vi "Load from File.vi"(5 "File Path (dialog)":path, 11 "Error In":errorcluster) -> (4 "Neural Network Out":T1={"Weigths"=[], "Last Layer Linear"=TRUE, "Add Bias Inputs"=TRUE, "# Inputs"=0, "# Output Neurons/Outputs"=0, "Inputs Scaling"={"X Scaling Vector"=[], "Y Scaling Vector"=[]}, "Outputs Scaling"={"X Scaling Vector"=[], "Y Scaling Vector"=[]}}, 6 "Used Path":path, 10 "Cancelled":bool, 15 "Error Out":errorcluster)   [LabVIEW 2013, in "Super Simple Neural Network.lvlib"]
doc: "This VI loads neural network from a file."
uses:
  Super Simple Neural Network.lvlib
  Types/Neural Network.ctl
  Types/2D Array.ctl
  Types/Scaling Info.ctl
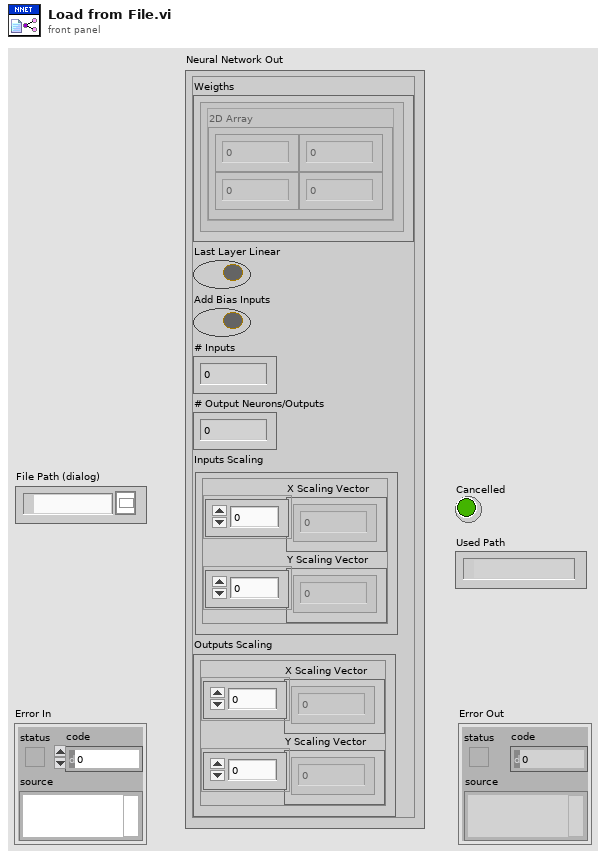
[diagram p1: front panel]
types:
  T1 = typedef "Super Simple Neural Network.lvlib/Neural Network.ctl" = cluster{"Weigths":T2[], "Last Layer Linear":bool, "Add Bias Inputs":bool, "# Inputs":u32, "# Output Neurons/Outputs":u32, "Inputs Scaling":T3, "Outputs Scaling":T3}
  T2 = typedef "Super Simple Neural Network.lvlib/2D Array.ctl" = cluster{"2D Array":dbl[][]}
  T3 = typedef "Super Simple Neural Network.lvlib/Scaling Info.ctl" = cluster{"X Scaling Vector":dbl[], "Y Scaling Vector":dbl[]}
  T4 = enum16{"open", "replace", "create", "open or create", "replace or create", "replace or create with confirmation"}
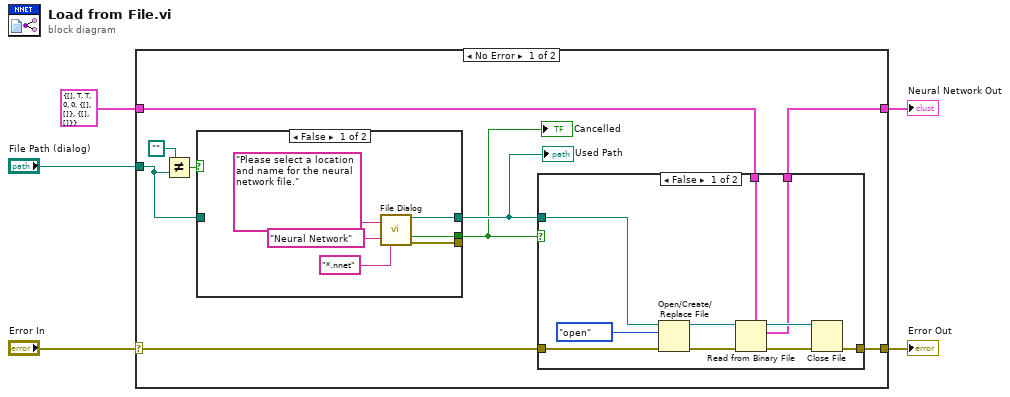
[diagram p0: block diagram]
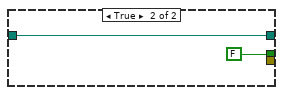
[diagram p3: hidden frame]
diagram:
  n1 = case shown="No Error" "Error In" {
    selector: "Error In" -> [w13 w36]
    tunnel: [w11 w36] -> w4
    tunnel: [w9 w35] -> w2
    tunnel: T1 {"Weigths"=[], "Last Layer Linear"=TRUE, "Add Bias Inputs"=TRUE, "# Inputs"=0, "# Output Neurons/Outputs"=0, "Inputs Scaling"={"X Scaling Vector"=[], "Y Scaling Vector"=[]}, "Outputs Scaling"={"X Scaling Vector"=[], "Y Scaling Vector"=[]}} ("Neural Network In") -> [w12 w35]
    tunnel: "File Path (dialog)" -> [w6 _]
    frame No Error {
      n2 = Not Equal?(x=path "", y=w6) -> (x != y?=w7:bool)
      n3 = case shown="False" w7 {
        tunnel: [w29 w34] -> w14
        tunnel: w6 -> [_ w34]
        tunnel: [w28 FALSE ("cancelled")] -> w10
        tunnel: [w27 _] -> _
        frame False {
          n4 = call "File Dialog"("prompt"="Please select a location and name for the neural network file.", "pattern (all files)"="*.nnet", "pattern label"="Neural Network") -> ("selected path"=w29:path, "cancelled"=w28:bool, "error out"=w27:errorcluster)  [unwired: 9 in, 1 out]
        }
        frame True {
        }
      }
      "Cancelled" <- w10
      "Used Path" <- w14
      n5 = case shown="False" w10 {
        tunnel: w14 -> [w24 _]
        tunnel: w13 -> [w21 w26]
        tunnel: w12 -> [w16 w25]
        tunnel: [w17 w26] -> w11
        tunnel: [w15 w25] -> w9
        frame False {
          n6 = Open/Create/Replace File(file path (use dialog)=w24, error in=w21, operation (0:open)=T4."open") -> (refnum out=w23:refnum<file>, error out=w20:errorcluster)  [unwired: 3 in, 1 out]
          n7 = Read from Binary File(5:w16, 8:w20, 11:w23) -> (0:w18:errorcluster, 2:w15:T1, 3:w19:refnum<file>)  [unwired: 3 in, 1 out]
          n8 = Close File(refnum=w19, error in=w18) -> (error out=w17:errorcluster)  [unwired: 1 out]
        }
        frame True {
        }
      }
    }
    frame Error {
    }
  }
  "Error Out" <- w4
  "Neural Network Out" <- w2
